vi "SubVI_MotorSimulation.vi"(7 "Input Voltage":dbl, 8 "Velocity Reading":dbl, 9 "dt [s]":dbl, 10 "Position Reading":dbl, 11 "System Parameters":cluster{"a1":dbl, "a0":dbl, "a2 ":dbl, "b":dbl}) -> (2 "Theta Out":dbl, 3 "Thetadot Out":dbl)   [LabVIEW 2022 SP3]
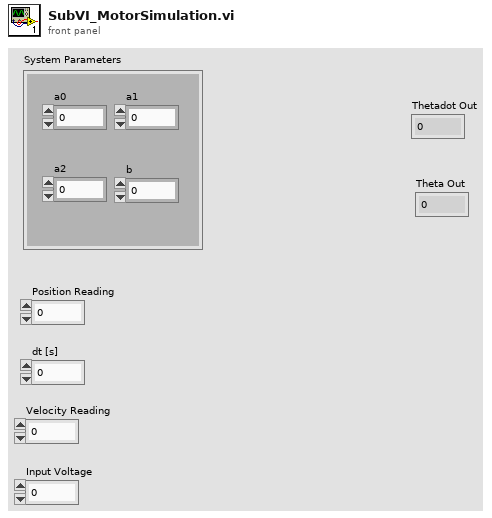
[diagram p1: front panel]
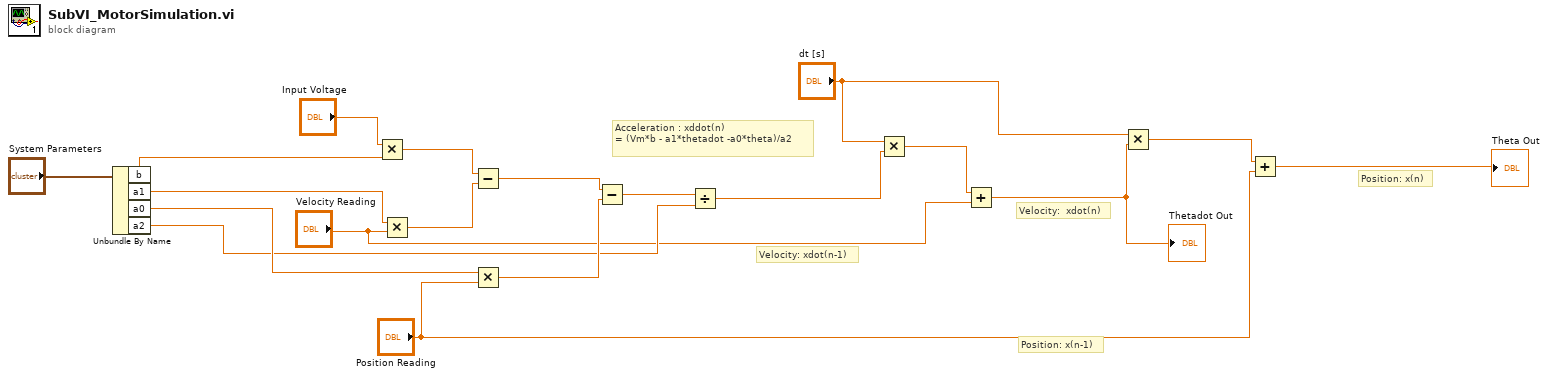
[diagram p0: block diagram]
diagram:
  # "Position: x(n)"
  # "Position: x(n-1)"
  # "Velocity:  xdot(n)"
  # "Velocity: xdot(n-1)"
  # "Acceleration : xddot(n) \n= (Vm*b - a1*thetadot -a0*theta)/a2"
  n1 = Unbundle By Name("System Parameters") -> ("b"=w17:dbl, "a1"=w16:dbl, "a0"=w12:dbl, "a2"=w9:dbl)
  n2 = Multiply(x="Input Voltage", y=w17) -> (x*y=w15:dbl)
  n3 = Multiply(x=w16, y="Velocity Reading") -> (x*y=w14:dbl)
  n4 = Subtract(x=w15, y=w14) -> (x-y=w13:dbl)
  n5 = Multiply(x=w12, y="Position Reading") -> (x*y=w11:dbl)
  n6 = Subtract(x=w13, y=w11) -> (x-y=w10:dbl)
  n7 = Divide(x=w10, y=w9) -> (x/y=w8:dbl)
  n8 = Multiply(x="dt [s]", y=w8) -> (x*y=w7:dbl)
  n9 = Add(x=w7, y="Velocity Reading") -> (x+y=w2:dbl)
  "Thetadot Out" <- w2
  n10 = Multiply(x="dt [s]", y=w2) -> (x*y=w4:dbl)
  n11 = Add(x=w4, y="Position Reading") -> (x+y=→"Theta Out":dbl)
